vi "Untitled 2.vi"(6 "ROI Descriptor":T2={"Global Rectangle"=[2791, 616, 3108, 922], "Contours"=[{"ID"=enum."External", "Type"=12, "Coordinates"=[2794, 619, 3105, 919, 359147]}]} {"Contours"."Type" items=["No Selection", "Point", "Line", "Rectangle", "Oval", "Polygon", "Freehand Region", "Annulus", "Unused2", "Unused3", "Broken Line", "Freehand Line", "Rotated Rectangle"]}, 9 "Matches (pixel)":T3(array[cluster]) {"Bounding Box"."y" format="%.2f"; "Bounding Box"."x" format="%.2f"; "Score" format="%.2f"; "Scale" format="%.2f"; "Angle" format="%.2f"; "Position"."y" format="%.2f"; "Position"."x" format="%.2f"}, 10 "Image Dst":T1, 11 "Image in":T1) -> (3 "Image Dst Out":T1)   [LabVIEW 2019]
uses:
  <vilib>/vision/Image Controls.llb/IMAQ Image.ctl
  <vilib>/vision/NI_Vision_Development_Module.lvlib
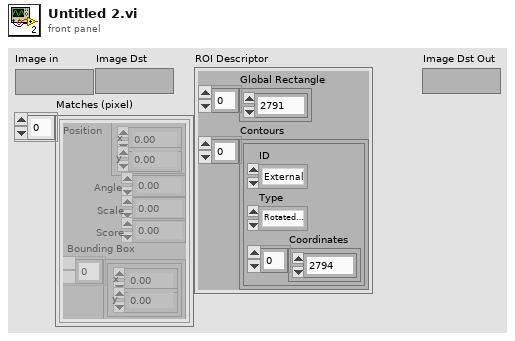
[diagram p1: front panel]
types:
  T1 = typedef "IMAQ Image.ctl" = refnum<image>
  T2 = cluster{"Global Rectangle":i32[], "Contours":cluster{"ID":enum32{"External", "Internal"}, "Type":u32, "Coordinates":i32[]}[]}
  T3 = cluster{"Position":cluster{"x":sgl, "y":sgl}, "Angle":sgl, "Scale":sgl, "Score":sgl, "Bounding Box":cluster{"x":sgl, "y":sgl}[]}[]
  T4 = cluster{"Origin":cluster{"X":sgl, "Y":sgl}, "Angle (deg)":sgl, "Axis Reference":u32}
  T5 = enum16{"Reset", "Update Coordinate System", "Get Coordinate System"}
  T6 = enum16{"Horizontal Motion", "Vertical Motion", "Horizontal and Vertical Motion", "Horizontal, Vertical and Angular Motion"}
  T7 = typedef "IMAQ Coordinate System" = cluster{"Reference System":cluster{"Origin":cluster{"X":sgl, "Y":sgl}, "Angle (deg)":sgl, "Axis Reference":u32}, "Measurement System":cluster{"Origin":cluster{"X":sgl, "Y":sgl}, "Angle (deg)":sgl, "Axis Reference":u32}}
  T8 = typedef "ROI Descriptor" = cluster{"Global Rectangle":i32[], "Contours":cluster{"ID":enum32{"External", "Internal"}, "Type":u32, "Coordinates":i32[]}[]}
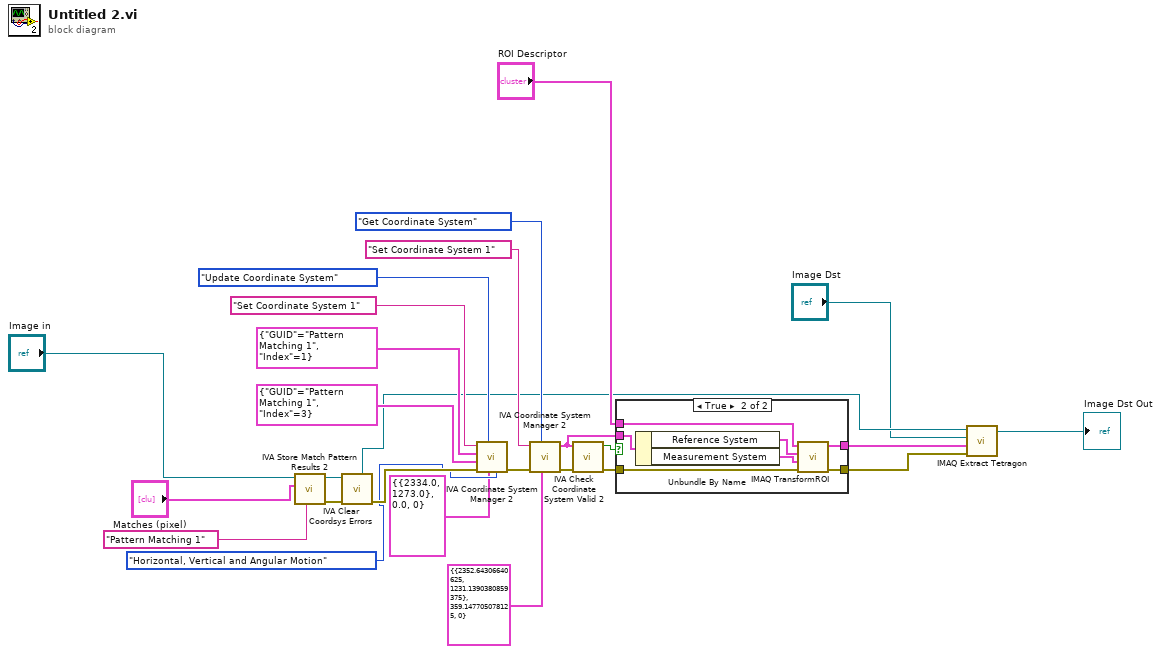
[diagram p0: block diagram]
diagram:
  n1 = call <vilib>:"IVA Store Match Pattern Results 2.vi"("Step Name"="Pattern Matching 1" ("GUID"), "Matches (pixel)"="Matches (pixel)", "Image in"="Image in") -> ("error out"=w25:errorcluster, "Image dup"=w4:T1)  [unwired: 3 in, 4 out]
  n2 = call <vilib>:"IVA Clear Coordsys Errors.vi"("error in (no error)"=w25) -> ("error out"=w24:errorcluster)  [unwired: 10 in]
  n3 = call <vilib>:"IVA Coordinate System Manager 2.vi"("Mode"=T6."Horizontal, Vertical and Angular Motion", "Reference System"=T4 {"Origin"={"X"=2334.0, "Y"=1273.0}, "Angle (deg)"=0.0, "Axis Reference"=0}, "Function"=T5."Update Coordinate System", "error in (no error)"=w24, "Angle ID"=cluster{"GUID":string, "Index":i32} {"GUID"="Pattern Matching 1", "Index"=3}, "Origin ID"=cluster{"GUID":string, "Index":i32} {"GUID"="Pattern Matching 1", "Index"=1}, "Coordinate System Name"="Set Coordinate System 1") -> ("error out"=w17:errorcluster)  [unwired: 4 out]
  n4 = call <vilib>:"IVA Coordinate System Manager 2.vi"("Reference System"=T4 {"Origin"={"X"=2352.643, "Y"=1231.139}, "Angle (deg)"=359.1477, "Axis Reference"=0}, "Function"=T5."Get Coordinate System", "error in (no error)"=w17, "Coordinate System Name"="Set Coordinate System 1") -> ("error out"=w7:errorcluster, "Coordinate System Out"=w6:T7)  [unwired: 3 in, 3 out]
  n5 = call <vilib>:"IVA Check Coordinate System Valid 2.vi"("error in (no error)"=w7, "Coordinate System"=w6) -> ("error out"=w8:errorcluster, "Valid?"=w9:bool)  [unwired: 8 out]
  n6 = case shown="True" w9 {
    tunnel: "ROI Descriptor" -> [w27 w34]
    tunnel: [w27 w31] -> w1
    tunnel: [w26 w30] -> w5
    tunnel: w6 -> [_ w29]
    tunnel: w8 -> [w26 w28]
    frame False {
    }
    frame True {
      n7 = Unbundle By Name(w29) -> ("Reference System"=w33:T4, "Measurement System"=w32:T4)
      n8 = call "IMAQ TransformROI"("error in (no error)"=w28, "New Reference"=w32, "Base Reference"=w33, "ROI Descriptor"=w34) -> ("error out"=w30:errorcluster, "ROI Descriptor out"=w31:T8)  [unwired: 6 out]
    }
  }
  n9 = call-poly "IMAQ Extract Tetragon"("error in (no error)"=w5, "ROI Descriptor"=w1, "Image Dst"="Image Dst", "Image Src"=w4) -> ("Image Dst Out"=→"Image Dst Out":T1)  [unwired: 6 in, 1 out]
